vi "Launch Config Dialog.vi"(8 "error in (no error)":errorcluster, 11 "Function in":refnum<class "Function.lvclass">) -> (0 "error out":errorcluster, 3 "Function out":refnum<class "Function.lvclass">)   [LabVIEW 2016, in "Function Actor.lvlib" / "Function.lvclass"]
uses:
  <userlib>/Common Components/Function Actor/Function.lvclass
  C:/Program Files (x86)/National Instruments/LabVIEW 2016/vi.lib/ActorFramework/Actor/Actor.lvclass
  <userlib>/Common Components/Function Actor/Function.lvclass/Function.ctl
  <vilib>/ActorFramework/Actor/Actor.lvclass/Actor.ctl
  <vilib>/ActorFramework/Message Enqueuer/Message Enqueuer.lvclass/Message Enqueuer.ctl
  <vilib>/ActorFramework/Message Enqueuer/Init from Existing Queue.vi
  <userlib>/Configuration Dialog Actor/Configuration.lvclass
  <vilib>/ActorFramework/Message Enqueuer/Message Enqueuer.lvclass
  <vilib>/ActorFramework/Actor/Actor.lvclass
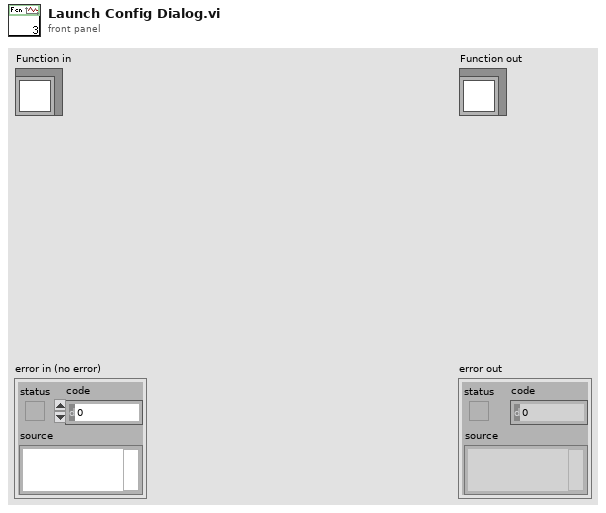
[diagram p1: front panel]
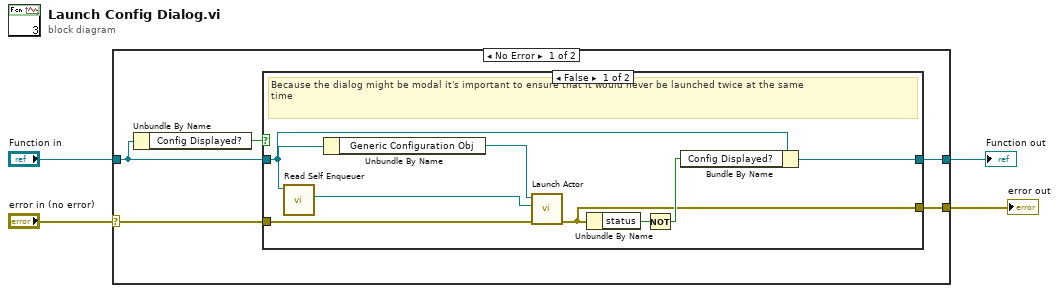
[diagram p0: block diagram]
diagram:
  n1 = case shown="No Error" "error in (no error)" {
    selector: "error in (no error)" -> [w5 w21]
    tunnel: [w8 w21] -> w3
    tunnel: [w9 w20] -> w4
    tunnel: "Function in" -> [w7 w20]
    frame No Error {
      n2 = Unbundle By Name(w7) -> ("Config Displayed?"=w6:bool)
      n3 = case shown="False" w6 {
        tunnel: [w15 w18] -> w9
        tunnel: [w11 w19] -> w8
        tunnel: w7 -> [w12 w18]
        tunnel: w5 -> [w13 w19]
        frame False {
          # "Because the dialog might be modal it's important to ensure that it would never be launched twice at the same\ntime"
          n4 = call <vilib>:"Read Self Enqueuer.vi"("Actor"=w12) -> ("Self Enqueuer"=w16:refnum<class "Message Enqueuer.lvclass">)  [unwired: 10 in]
          n5 = Unbundle By Name(w12) -> ("Generic Configuration Obj"=w17:refnum<class "Configuration.lvclass">)
          n6 = call <vilib>:"Launch Actor.vi"("error in (no error)"=w13, "Actor-to-Caller Enqueuer"=w16, "Actor"=w17) -> ("error out"=w11:errorcluster)  [unwired: 7 in, 1 out]
          n7 = Unbundle By Name(w11) -> ("status"=w10:bool)
          n8 = Not(x=w10) -> (.not. x?=w14:bool)
          n9 = Bundle By Name(cluster=w12, "Config Displayed?"=w14) -> (w15:refnum<class "Function.lvclass">)
        }
        frame True {
        }
      }
    }
    frame Error {
    }
  }
  "error out" <- w3
  "Function out" <- w4
